vi "Clear Nexteer NTCs.vi"(6 "error in":errorcluster, 8 "MaxRead":i32, 9 "Channel in":u16) -> (0 "error out":errorcluster, 1 "Messages":T1(array[cluster]), 2 "Pass":bool, 3 "Channel out":u16)   [LabVIEW 2023]
uses:
  Communication/PCAN2023/PCAN API.lvlib
  f7b1ebe6-23a2-4c52-841e-065e5075a79d.vi
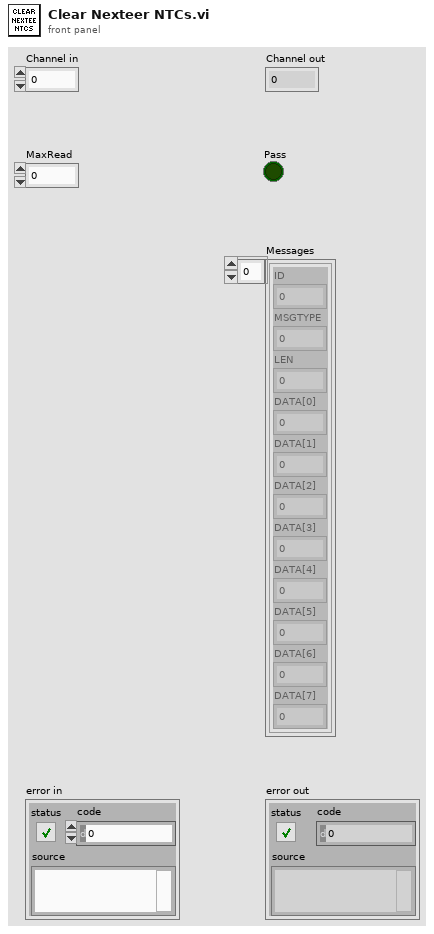
[diagram p1: front panel]
types:
  T1 = cluster{"ID":u32, "MSGTYPE":u8, "LEN":u8, "DATA[0]":u8, "DATA[1]":u8, "DATA[2]":u8, "DATA[3]":u8, "DATA[4]":u8, "DATA[5]":u8, "DATA[6]":u8, "DATA[7]":u8}[]
  T2 = cluster{"ID":u32, "MSGTYPE":u8, "LEN":u8, "DATA[0]":u8, "DATA[1]":u8, "DATA[2]":u8, "DATA[3]":u8, "DATA[4]":u8, "DATA[5]":u8, "DATA[6]":u8, "DATA[7]":u8}
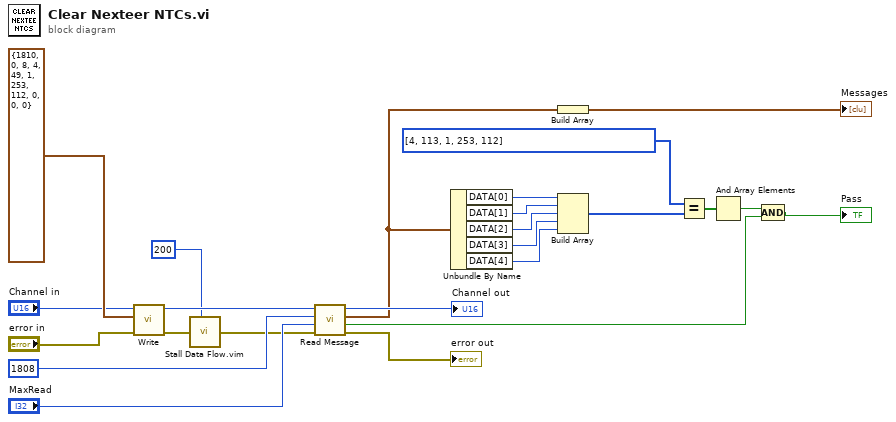
[diagram p0: block diagram]
diagram:
  n1 = call "Write.vi"("error in"="error in", "MessageBuffer"=T2 {"ID"=1810, "MSGTYPE"=0, "LEN"=8, "DATA[0]"=4, "DATA[1]"=49, "DATA[2]"=1, "DATA[3]"=253, "DATA[4]"=112, "DATA[5]"=0, "DATA[6]"=0, "DATA[7]"=0}, "Channel"="Channel in") -> ("error out"=w8:errorcluster, "Channel out"=w10:u16)  [unwired: 5 in, 2 out]
  n2 = call "Stall Data Flow.vim"("value in"=w8, "milliseconds to wait"=u32 200) -> ("value out"=w2:errorcluster)  [unwired: 1 out]
  n3 = call "Read Message.vi"("error in"=w2, "MaxRead"="MaxRead", "ID"=u32 1808, "Channel in"=w10) -> ("error out"=→"error out":errorcluster, "Passed"=w5:bool, "Last Message"=w6:T2, "Channel out"=→"Channel out":u16)  [unwired: 3 in, 1 out]
  n4 = Unbundle By Name(w6) -> ("DATA[0]"=w19:u8, "DATA[1]"=w18:u8, "DATA[2]"=w17:u8, "DATA[3]"=w16:u8, "DATA[4]"=w15:u8)
  n5 = Build Array(w6) -> (→"Messages":T1)
  n6 = Build Array(w19, w18, w17, w16, w15) -> (w13:u8[])
  n7 = Equal?(x=u8[] [4, 113, 1, 253, 112], y=w13) -> (x = y?=w21:bool[])
  n8 = And Array Elements(Boolean array=w21) -> (logical AND=w12:bool)
  n9 = Compound Arithmetic op=AND(w12, w5) -> (→"Pass":bool)
